vi "Type Cast Node.vi"(8 "error in":errorcluster, 11 "Node in":refnum<class "Node.lvclass">) -> (0 "error out":errorcluster, 3 "Node out":refnum<class "Node.lvclass">)   [LabVIEW 2014, in "Node.lvclass"]
uses:
  Node.lvclass
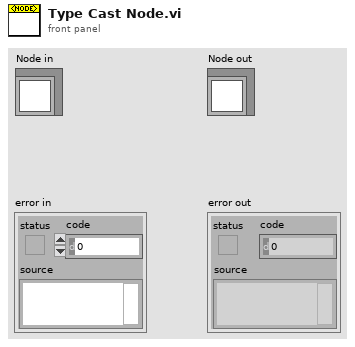
[diagram p1: front panel]
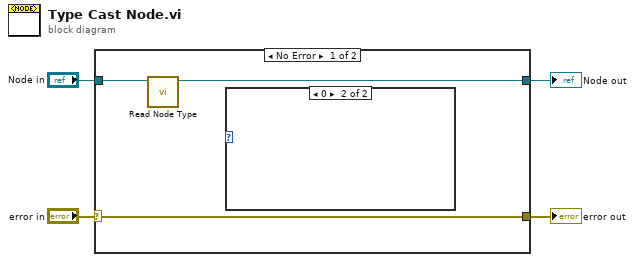
[diagram p0: block diagram]
diagram:
  n1 = case shown="No Error" "error in" {
    selector: "error in" -> [w6 w9]
    tunnel: [w6 w9] -> w3
    tunnel: [w5 w8] -> w1
    tunnel: "Node in" -> [w7 w8]
    frame No Error {
      n2 = call-dynamic "Read Node Type.vi"("Node in"=w7) -> ("Node out"=w5:refnum<class "Node.lvclass">)  [unwired: 8 in, 2 out]
      n3 = case shown="0" {
        selector: _ -> [_ _]
        frame Default {
        }
        frame 0 {
        }
      }
    }
    frame Error {
    }
  }
  "error out" <- w3
  "Node out" <- w1
